vi "Help1.vi"() -> ()   [LabVIEW 2011]
panel:
  in  "选项卡控件":enum32{"修正记录", "版本历史"}(tab)
  out "字符串":string
  out "字符串 2":string
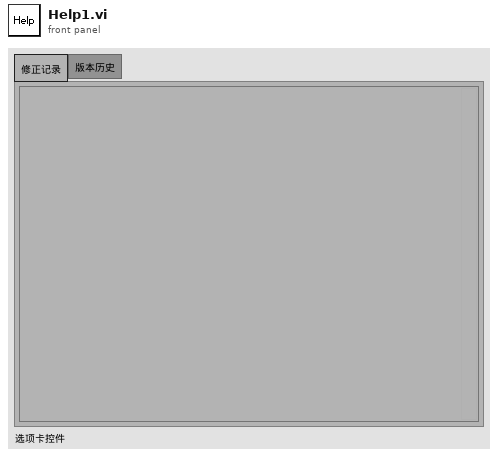
[diagram p1: front panel]
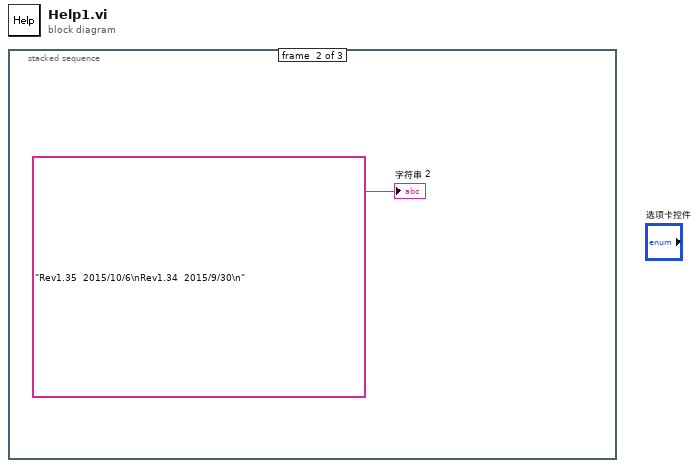
[diagram p0: block diagram]
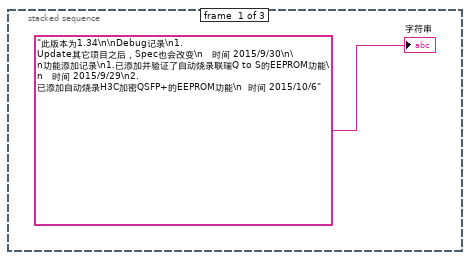
[diagram p2: hidden frame]
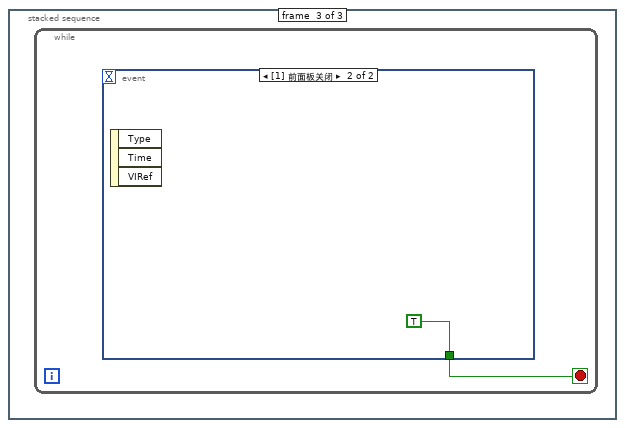
[diagram p3: hidden frame]
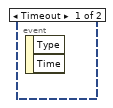
[diagram p4: hidden frame]
diagram:
  n1 = stacked-sequence {
    frame #0 {
      "字符串" <- "此版本为1.34\n\nDebug记录\n1.Update其它项目之后，Spec也会改变\n   时间 2015/9/30\n\n功能添加记录\n1.已添加并验证了自动烧录联瑞Q to S的EEPROM功能\n   时间 2015/9/29\n2.已添加自动烧录H3C加密QSFP+的EEPROM功能\n  时间 2015/10/6" ("字符串")
    }
    frame #1 {
      "字符串 2" <- "Rev1.35  2015/10/6\nRev1.34  2015/9/30\n" ("字符串 2")
    }
    frame #2 {
      n2 = while {
        stop <- w3 stop-if-true
        n3 = event shown="[1] 前面板关闭" {
          selector: _ -> [_ _]
          dyn-events: _ -> [_ _]
          timeout: _ -> [_ _]
          tunnel: [_ TRUE] -> w3
          event Timeout {
            n4 = event-data() -> ()  [unwired: 1 in, 2 out]
          }
          event Panel Close {
            n5 = event-data() -> ()  [unwired: 1 in, 3 out]
          }
        }
      }
    }
  }
